vi "User Plugin.vi"(5 "Initialize":bool, 8 "error in (no error)":errorcluster, 10 "ParamValues":sgl[](array[numeric]), 11 "DSI Reference":refnum<class "DCM-DSI-UserRPCExample.lvclass">) -> (0 "error out":errorcluster, 3 "DSI Reference":refnum<class "DCM-DSI-UserRPCExample.lvclass">, 4 "Results":T1[](array[typedef]), 6 "ParamNames":string[](array[string]))   [LabVIEW 2016, in "DCM-DSI-UserRPCExample.lvclass"]
uses:
  DCM-DSI-UserRPCExample.lvclass
  D:/PCG/Products/DCM/Software/DCM-DSI/Classes/DCM-DSI/DCM-DSI.lvclass
  Shared/Typedefs/UserParameter.ctl
  <vilib>/Powertrain Controls/Device Drivers/DCM/HH/RT/Setup.ctl
  <vilib>/Powertrain Controls/Device Drivers/DCM/HH/FPGA/Mode.ctl
  <vilib>/Powertrain Controls/Device Drivers/DCM/Rev0/FPGA/Digital Channel.ctl
  <vilib>/Powertrain Controls/Device Drivers/DCM/HH/RT/Angle Control.ctl
  DCM-DSI/Read HH Command.vi
  DCM-DSI/Read Channels.vi
  DCM-DSI/Read dt.vi
  DCM-DSI/Write HH Command.vi
  <vilib>/Powertrain Controls/Device Drivers/DCM/HH/FPGA/DCM - FPGA - HH.lvlib
  <vilib>/Powertrain Controls/Device Drivers/DCM/Rev0/FPGA/DCM - FPGA.lvlib
  <vilib>/Powertrain Controls/Device Drivers/DCM/HH/RT/DCM - RT - HH.lvlib
  Shared/DSI-Shared.lvlib
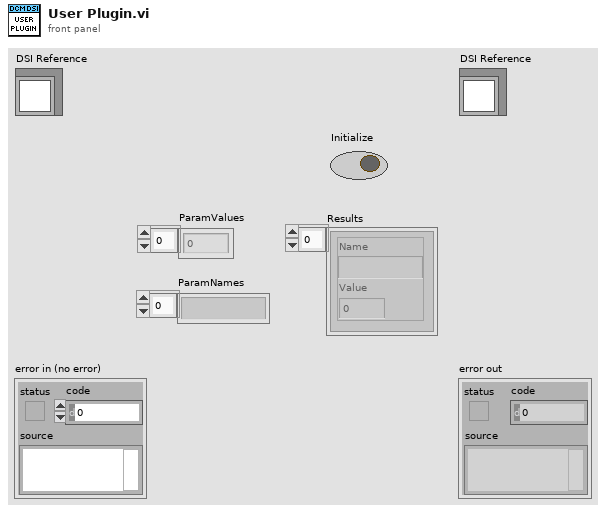
[diagram p1: front panel]
types:
  T1 = typedef "DSI-Shared.lvlib/UserParameter.ctl" = cluster{"Name":string, "Value":dbl}
  T2 = typedef "DCM - FPGA - HH.lvlib/Mode.ctl" = enum8{"Off", "Direct", "Pulse Width Modulation", "Engine Position Tracking"}
  T3 = typedef "DCM - RT - HH.lvlib/Setup.ctl" = cluster{"Mode":T2, "Digital Input":T4, "Polarity":bool, "Frequency [Hz]":sgl, "Duty Cycle [%]":sgl, "TDC Offset [CAD]":sgl, "Window Start [DBTDC]":sgl, "Window End [DBTDC]":sgl, "Angles":T5[], "Skip Fire":bool, "Skip Fire Index":u8}
  T4 = typedef "DCM - FPGA.lvlib/Digital Channel.ctl" = enum8{"Unused", "User OS", "Diff IO 1", "Diff IO 2", "Diff IO 3", "Diff IO 4", "Diff IO 5", "Diff IO 6", "Diff IO 7", "Diff IO 8", "Aux 1", "Aux 2", "Aux 3", "Aux 4", "Aux 5", "Aux 6", "Aux 7", "Aux 8", "Aux 9", "Aux 10", "Aux 11", "Aux 12", "Aux 13", "Aux 14", "Aux 15", "Aux 16"}
  T5 = typedef "DCM - RT - HH.lvlib/Angle Control.ctl" = cluster{"Enable":bool, "Location [DBTDC]":sgl, "Duration [s]":sgl}
  T6 = typedef "DSI-Shared.lvlib/Engine-Channel.ctl" = cluster{"Name":string, "Unit":string, "Value":sgl}
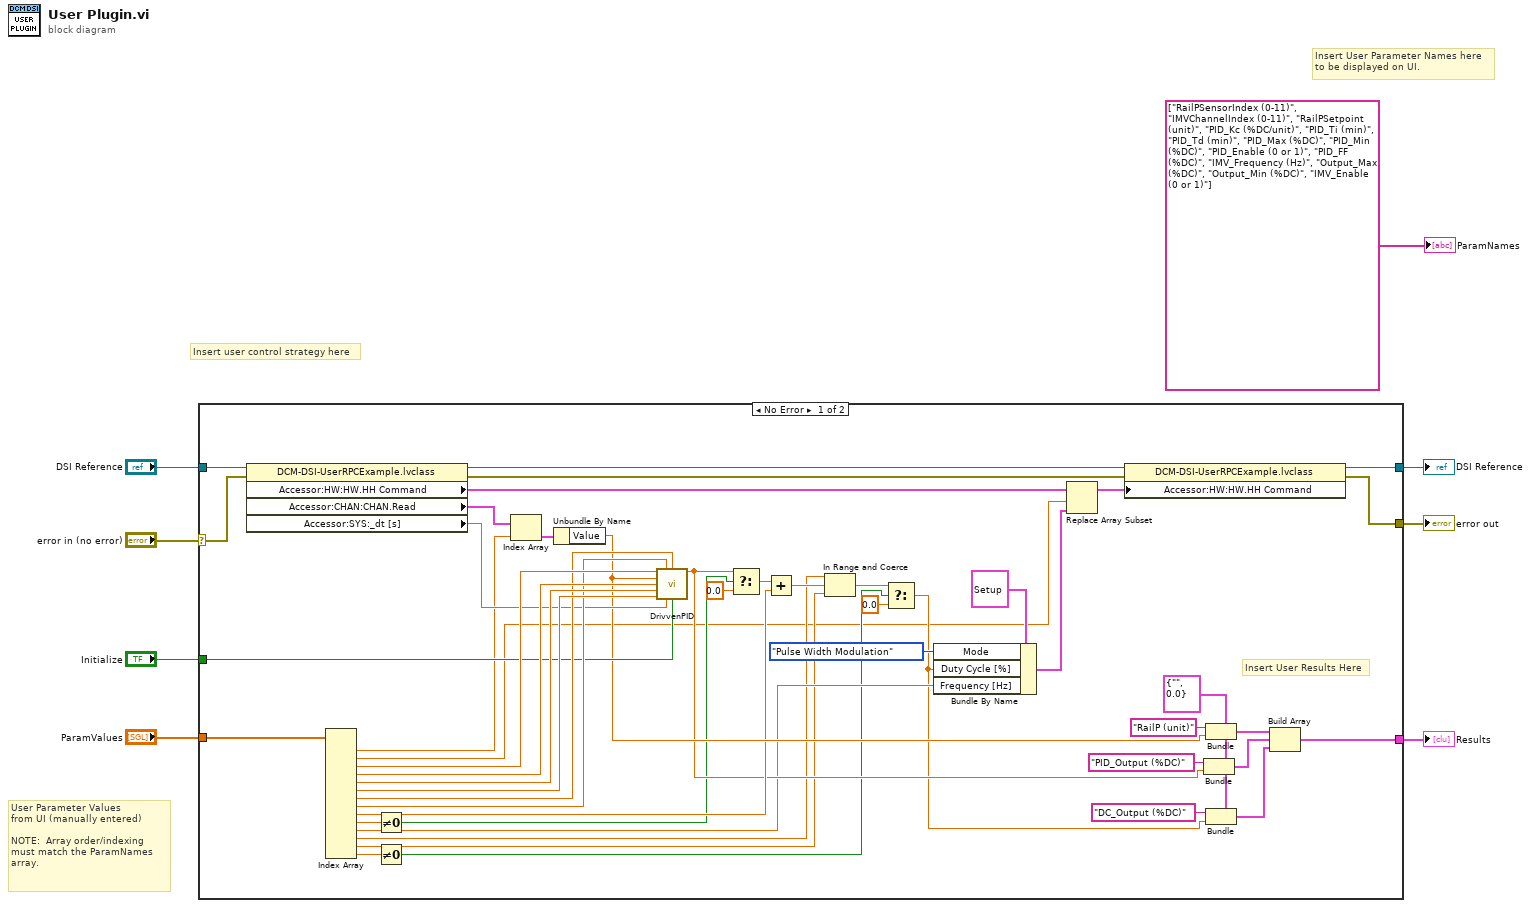
[diagram p0: block diagram]
diagram:
  # "User Parameter Values\nfrom UI (manually entered)\n\nNOTE:  Array order/indexing\nmust match the ParamNames\narray."
  # "Insert user control strategy here"
  # "Insert User Parameter Names here\nto be displayed on UI."
  n1 = case shown="No Error" "error in (no error)" {
    selector: "error in (no error)" -> [w56 w58]
    tunnel: [w55 w58] -> w7
    tunnel: [w53 w57] -> w5
    tunnel: "DSI Reference" -> [w54 w57]
    tunnel: "Initialize" -> [w36 _]
    tunnel: "ParamValues" -> [w52 _]
    tunnel: [w51 _] -> w2
    frame No Error {
      w18 = T1 {"Name"="", "Value"=0.0} ("User Parameter")
      # "Insert User Results Here"
      n2 = property class="DCM-DSI-UserRPCExample.lvclass"(reference=w54, error in=w56) -> (reference out=w45:refnum<class "DCM-DSI-UserRPCExample.lvclass">, error out=w46:errorcluster, "Accessor:HW:HW.HH Command"=w12:T3[], "Accessor:CHAN:CHAN.Read"=w13:T6[], "Accessor:SYS:_dt [s]"=w37:sgl)
      n3 = Index Array(array=w52) -> (element #1=w22:sgl, element #2=w9:sgl, element #3=w44:sgl, element #4=w42:sgl, element #5=w41:sgl, element #6=w40:sgl, element #7=w39:sgl, element #8=w38:sgl, element #9=w34:sgl, element #10=w33:sgl, element #11=w27:sgl, element #12=w15:sgl, element #13=w14:sgl, element #14=w16:sgl)  [unwired: 14 in]
      n4 = Not Equal To 0?(x=w33) -> (x != 0?=w29:bool)
      n5 = Not Equal To 0?(x=w16) -> (x != 0?=w24:bool)
      n6 = Index Array(array=w13, index=w22) -> (element=w43:T6)
      n7 = Unbundle By Name(w43) -> ("Value"=w35:sgl)
      n8 = call <vilib>:"DrivvenPID.vi"("Setpoint"=w44, "OutputLow"=w38, "OutputHigh"=w39, "ProcessVariable"=w35, "ProportionalGain (Kc)"=w42, "IntegralTime (Ti, min)"=w41, "DerivativeTime (Td, min)"=w40, "dt (s)"=w37, "Reinitialize? (F)"=w36) -> ("Output"=w31:sgl)  [unwired: 1 in, 5 out]
      n9 = Select(t=w31, s=w29, f=sgl 0.0) -> (s? t:f=w32:sgl)
      n10 = Add(x=w32, y=w34) -> (x+y=w25:sgl)
      n11 = In Range and Coerce(upper limit=w15, x=w25, lower limit=w14) -> (coerced(x)=w17:sgl)  [unwired: 1 out]
      n12 = Select(t=w17, s=w24, f=sgl 0.0) -> (s? t:f=w20:sgl)
      n13 = Bundle By Name(cluster=T3 {"Mode"=enum."Off", "Digital Input"=enum."Unused", "Polarity"=FALSE, "Frequency [Hz]"=0.0, "Duty Cycle [%]"=0.0, "TDC Offset [CAD]"=0.0, "Window Start [DBTDC]"=0.0, "Window End [DBTDC]"=0.0, "Angles"=[{"Enable"=FALSE, "Location [DBTDC]"=0.0, "Duration [s]"=0.0}, {"Enable"=FALSE, "Location [DBTDC]"=0.0, "Duration [s]"=0.0}, {"Enable"=FALSE, "Location [DBTDC]"=0.0, "Duration [s]"=0.0}, {"Enable"=FALSE, "Location [DBTDC]"=0.0, "Duration [s]"=0.0}], "Skip Fire"=FALSE, "Skip Fire Index"=0} ("HH Command"), "Mode"=Mode."Pulse Width Modulation", "Duty Cycle [%]"=w20, "Frequency [Hz]"=w27) -> (w10:T3)
      n14 = Replace Array Subset(array=w12, new element=w10, index=w9) -> (w11:T3[])
      n15 = property class="DCM-DSI-UserRPCExample.lvclass"(reference=w45, error in=w46, "Accessor:HW:HW.HH Command"=w11) -> (reference out=w53:refnum<class "DCM-DSI-UserRPCExample.lvclass">, error out=w55:errorcluster)
      n16 = Bundle(cluster=w18, "Name"="PID_Output (%DC)", "Value"=w31) -> (w49:T1)
      n17 = Bundle(cluster=w18, "Name"="RailP (unit)", "Value"=w35) -> (w47:T1)
      n18 = Bundle(cluster=w18, "Name"="DC_Output (%DC)", "Value"=w20) -> (w19:T1)
      n19 = Build Array(w47, w49, w19) -> (w51:T1[])
    }
    frame Error {
    }
  }
  "error out" <- w7
  "DSI Reference" <- w5
  "Results" <- w2
  "ParamNames" <- string[] ["RailPSensorIndex (0-11)", "IMVChannelIndex (0-11)", "RailPSetpoint (unit)", "PID_Kc (%DC/unit)", "PID_Ti (min)", "PID_Td (min)", "PID_Max (%DC)", "PID_Min (%DC)", "PID_Enable (0 or 1)", "PID_FF (%DC)", "IMV_Frequency (Hz)", "Output_Max (%DC)", "Output_Min (%DC)", "IMV_Enable (0 or 1)"] ("ParamNames")
